vi "Restart ADB Server.vi"(0 "adb location":string, 1 "error in":errorcluster) -> (2 "standard output":string, 3 "standard error":string, 4 "error out":errorcluster)   [LabVIEW 2016]
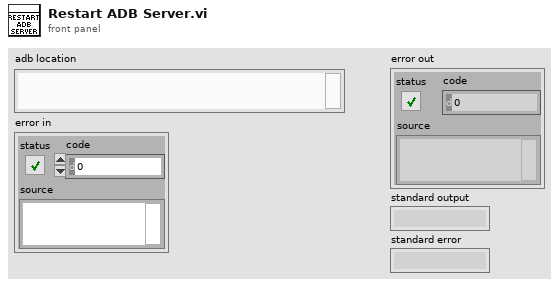
[diagram p1: front panel]
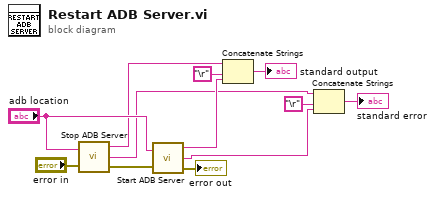
[diagram p0: block diagram]
diagram:
  n1 = call "Stop ADB Server.vi"("adb location"="adb location", "error in"="error in") -> ("standard output"=w8:string, "standard error"=w3:string, "error out"=w9:errorcluster)
  n2 = call "Start ADB Server.vi"("adb location"="adb location", "error in"=w9) -> ("standard output"=w7:string, "standard error"=w2:string, "error out"=→"error out":errorcluster)
  n3 = Concatenate Strings(w8, "\r", w7) -> (→"standard output":string)
  n4 = Concatenate Strings(w3, "\r", w2) -> (→"standard error":string)
